vi "wrap error metadata mini.vi"(8 "error in (no error)":errorcluster, 10 "state name":string, 11 "task name":string) -> (0 "error out":errorcluster)   [LabVIEW 2024, in "Error Wrapper.lvlib"]
doc: "Description:\nThis VI generates an extended error metadata cluster (Error_Metadata) that combines the original error with contextual information such as task name, state name, event name, calling VI, timestamp, and additional custom info.\n\nUsage:\nCall this VI from any state or task within a QMH (Queued Message Handler) architecture when an error occurs. Provide the current task, state, and event names, along with any optional notes or extra context. The VI validates and formats the inputs, enriches the 'source' field of the original error, and returns a complete metadata cluster for logging or centralized error handling.\n\nInputs:\n- error in: The original LabVIEW error cluster.\n- task name, state name.\n\nOutputs:\n- error out: The same error, with a modified source field for improved traceability.\n\nNotes:\n- Framework-agnostic: can be used with QMH, DQMH, Actor Framework, or custom architectures.\n- Especially useful for error routing to a central Error Handler loop.\n- Designed for scalability and readability in large applications."
uses:
  Error Wrapper.lvlib
  error field names.ctl
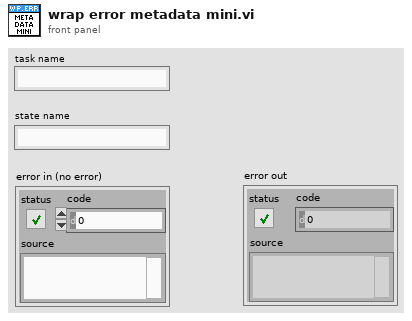
[diagram p1: front panel]
types:
  T1 = typedef "Error Wrapper.lvlib/error field names.ctl" = enum32{"TASK NAME", "STATE NAME", "EVENT NAME", "ADDITIONAL INFO"}
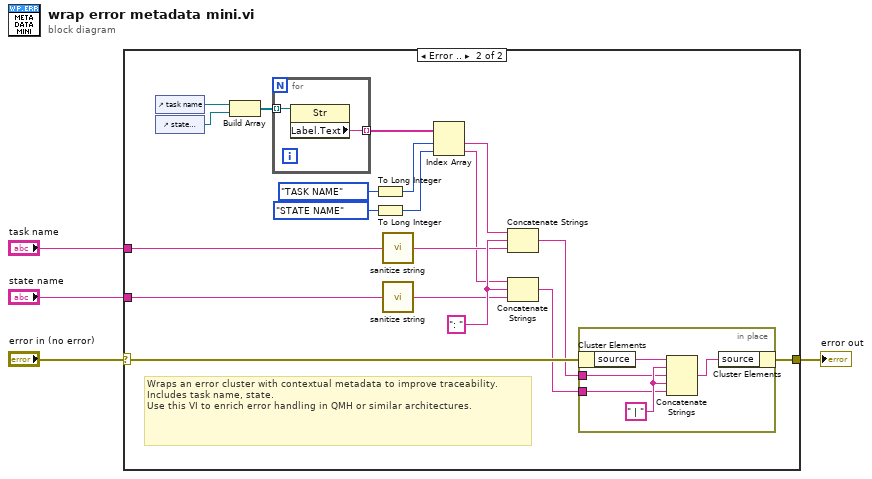
[diagram p0: block diagram]
diagram:
  n1 = case shown="Error .." "error in (no error)" {
    selector: "error in (no error)" -> [w5 w10]
    tunnel: "task name" -> [_ w22]
    tunnel: "state name" -> [_ w21]
    tunnel: [w5 w6] -> w1
    frame No Error {
    }
    frame Error {
      w24 = ": "
      # "Wraps an error cluster with contextual metadata to improve traceability.\nIncludes task name, state.\nUse this VI to enrich error handling in QMH or similar architectures."
      n2 = control-ref of="task name"() -> (w19:refnum<vi>)
      n3 = control-ref of="state name"() -> (w18:refnum<vi>)
      n4 = Build Array(w19, w18) -> (w17:refnum<vi>[])
      n5 = for {
        tunnel: w17 -> [w31] mode=indexing
        tunnel: [w30] -> w16 mode=indexing
        n6 = property on="Property Node" class="Str"(reference=w31) -> ("Label.Text"=w30:string)  [unwired: 1 in, 2 out]
      }
      n7 = To Long Integer(number=error_field_names."TASK NAME") -> (32bit integer=w13:i32)
      n8 = To Long Integer(number=error_field_names."STATE NAME") -> (32bit integer=w12:i32)
      n9 = call "sanitize string.vi"("string in"=w22) -> ("validated string"=w23:string)  [unwired: 4 in]
      n10 = call "sanitize string.vi"("string in"=w21) -> ("validated string"=w20:string)  [unwired: 4 in]
      n11 = Index Array(array=w16, index #1=w13, index #2=w12) -> (element #1=w7:string, element #2=w15:string)
      n12 = Concatenate Strings(w7, w24, w23) -> (w9:string)
      n13 = Concatenate Strings(w15, w24, w20) -> (w8:string)
      n14 = in-place "In Place Element Structure" {
        in-place-border: w9 -> [w27]
        in-place-border: w8 -> [w26]
        w28 = " | "
        n15 = in-place-cluster #1(w10) -> ("source"=w29:string)
        n16 = Concatenate Strings(w29, w28, w27, w28, w26) -> (w25:string)
        n17 = in-place-cluster #1("source"=w25) -> (w6:errorcluster)
      }
    }
  }
  "error out" <- w1
